vi "Framework Performance.Get Tx Duration.vi"(8 "error in (no error)":errorcluster, 11 "Framework Performance in":refnum<class "Framework Performance.lvclass">) -> (0 "error out":errorcluster, 2 "tx duration":u32 format="%d us", 3 "Framework Performance out":refnum<class "Framework Performance.lvclass">)   [LabVIEW 2017, in "DSF Core.lvlib" / "Framework Performance.lvclass"]
uses:
  Framework Performance.lvclass
  Framework Performance.lvclass/Framework Performance.ctl
  <vilib>/NI/Memory Manager/Classes/Pointer/Memory.Pointer.lvclass/Memory.Pointer.ctl
  <vilib>/NI/Memory Manager/Classes/Pointer/Memory.Pointer.Read.0D.U32.vi
  <vilib>/NI/Memory Manager/Classes/Pointer/Memory.Pointer.Read.No Check.0D.U32.vi
  <vilib>/NI/Memory Manager/Classes/Pointer/Memory.Pointer.Parameter Check.Null Pointer.vi
  <vilib>/NI/Memory Manager/Classes/Pointer/Memory.Pointer.Parameter Check.Subset.vi
  <vilib>/NI/Memory Manager/Classes/Pointer/Memory.Pointer.Get Address.vi
  <vilib>/NI/Memory Manager/Classes/Pointer/Memory.Pointer.Errors.vi
  <vilib>/NI/Memory Manager/Classes/Pointer/Memory.Pointer.Errors.Null Pointer.vi
  <vilib>/NI/Memory Manager/Classes/Pointer/Memory.Pointer.Errors.Out of Bounds.vi
  <vilib>/NI/Memory Manager/Classes/Pointer/Memory.Pointer.Get Size.vi
  <vilib>/NI/Memory Manager/Classes/Pointer/Memory.Pointer.Errors.Create Error.vi
  <vilib>/NI/Memory Manager/VIs/Source.Write.String.vi
  <vilib>/NI/Memory Manager/Classes/Pointer/Memory.Pointer.Errors.Write Pointer Size.vi
  <vilib>/NI/Memory Manager/VIs/Source.Write.Scalar.Base10.vi
  <vilib>/NI/Memory Manager/VIs/Source.Write.Scalar.Base10 (U64).vi
  <vilib>/NI/Memory Manager/VIs/New Error Cluster Constant.vi
  <vilib>/NI/Memory Manager/VIs/New Error Cluster Constant (512B).vi
  <vilib>/NI/Memory Manager/VIs/Error Cluster.Set Status.vi
  <vilib>/NI/Memory Manager/VIs/Error Cluster.Set Code.vi
  <vilib>/NI/Memory Manager/VIs/Error Cluster.Set VI Source.vi
  <vilib>/NI/Memory Manager/Constants/Memory.Constants.vi
  <vilib>/NI/Memory Manager/Constants/Memory.Constants.Library Name.vi
  <vilib>/NI/Memory Manager/Classes/Pointer/Memory.Pointer.Errors.Get Info.vi
  <vilib>/NI/Memory Manager/Classes/Pointer/Memory.Pointer.lvclass
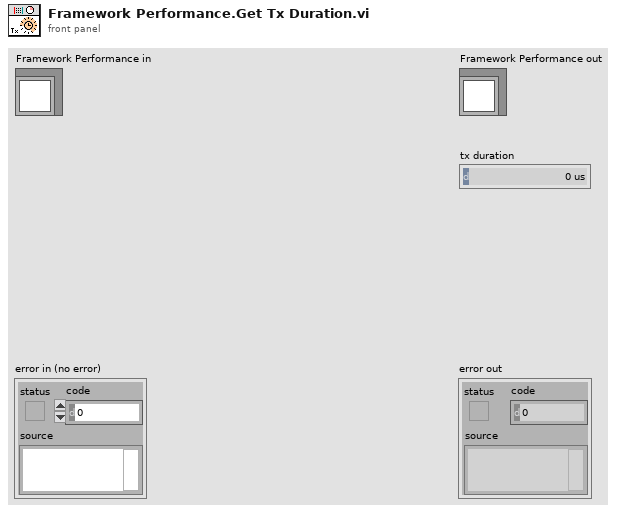
[diagram p1: front panel]
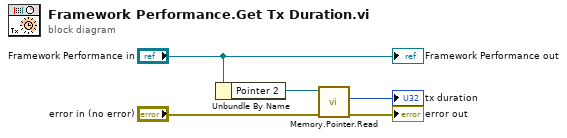
[diagram p0: block diagram]
diagram:
  n1 = Unbundle By Name("Framework Performance in") -> ("Pointer 2"=w5:refnum<class "Memory.Pointer.lvclass">)
  n2 = call-poly <vilib>:"Memory.Pointer.Read.vi"("error in (no error)"="error in (no error)", "Pointer in"=w5) -> ("error out"=→"error out":errorcluster, "value out"=→"tx duration":u32)  [unwired: 6 in, 2 out]
  "Framework Performance out" <- "Framework Performance in"
